vi "Dashboard Main.vi"() -> ()   [LabVIEW 2014]
uses:
  <vilib>/event_ctls.llb/eventvkey.ctl
  <vilib>/Rock Robotics/WPI/Dashboard/WPI_DashboardLogging Global.vi
  <vilib>/Utility/config.llb/Write Key (String).vi
  <vilib>/Utility/config.llb/Write Key (I32).vi
  <vilib>/Utility/config.llb/NI_LVConfig.lvlib
panel:
  in  "TCP":refnum<k5>
  in  "Rec Mode":enum32{"Stop", "Record", "Playback"}(radio)
  in  "Vision":u16(ring) items=["Camera Off", "USB Camera SW", "USB Camera HW", "IP Camera"]
  out "Camera IP":string
  out "Image Message":string="Timeout in Camera Communications"
  in  "Dashboard Tab":T1(tab)
  in  "Camera Settings":T2={"Frame Rate"=30, "Compression"=30, "Size"=1} {"Frame Rate" scale=1.0..30.0; "Size" items=["640x480", "320x240", "160x120"]}
  out "MotorChart R":cluster{"Numeric":dbl, "Numeric":dbl}(graph)
  out "MotorChart L":T3(graph)
  out "MotorSliders R":cluster{"MotorSlide1":dbl, "MotorSlide2":dbl} {"MotorSlide2" scale=-1.0..1.0 scale format="%#_2e"; "MotorSlide1" scale=-1.0..1.0 scale format="%#_2e"}
  out "MotorSliders L":T4 {"MotorSlide4 2" scale=0.0..14.0 scale format="%#_2e"; "MotorSlide2" scale=-1.0..1.0 scale format="%#_2e"; "MotorSlide1" scale=-1.0..1.0 scale format="%#_2e"}
  out "Mode":T5(ring)=enum."Auto Disabled"
  in  "DB Camera Config":bool
  out "fps":dbl format="%#.1g"
  out "Mbps":dbl format="%#.1g"
  out "Mbps 2":bool
  in  "DB/String 9":string
  in  "DB/String 8":string
  in  "DB/String 7":string
  in  "DB/String 6":string
  in  "DB/String 5":string
  in  "DB/String 4":string
  in  "DB/String 3":string
  in  "DB/String 2":string
  in  "DB/String 1":string
  in  "DB/String 0":string
  in  "DB/Slider 0":dbl(slide) scale=0.0..5.0
  in  "DB/Slider 1":dbl(slide) scale=0.0..5.0
  in  "DB/Slider 2":dbl(slide) scale=0.0..5.0
  in  "DB/Slider 3":dbl(slide) scale=0.0..5.0
  out "DB/LED 3":bool
  out "DB/LED 2":bool
  out "DB/LED 1":bool
  out "DB/LED 0":bool
  in  "DB/Button 3":bool
  in  "DB/Button 2":bool
  in  "DB/Button 1":bool
  in  "DB/Button 0":bool caption="New Name"
  in  "Auto Selection":string(combo)
  in  "Test Slider":dbl(slide) scale=0.0..100.0 scale format="%#_3g"
  in  "On/Off":bool caption="Solenoid"
  in  "Test Name":u16(ring) items=["Select the test to run...", "Example Test", "-------------------------------", "List of tests is built in robot code.", "Replace with your own automated tests."]
  in  "Test Tree":string(tree)
  in  "Motor":cluster{"Value":dbl, "Enable":bool} {"Value" scale=-1.0..1.0 scale format="%#_3g"}
  out "Progress":T6 {"Test Progress" scale=0.0..100.0}
  in  "Rev/Fwd":cluster{"Forward":bool, "Reverse":bool}
  in  "Test Ring":u16(ring) items=["Monochrome", "Color"]
  in  "Listbox":i32(listbox)
  out "Tree":string(tree)
  out "Camera Image":T7(plugin-control)
  out "Boolean":bool
  # "Left"
  # "Front"
  # "Right"
  # "Battery"
  # "This tab is a great place for autonomous settings and robot-specific values.\nPlace controls and indicators inside this tab and match name to\nDashboard Variables on robot. You can also delete this comment."
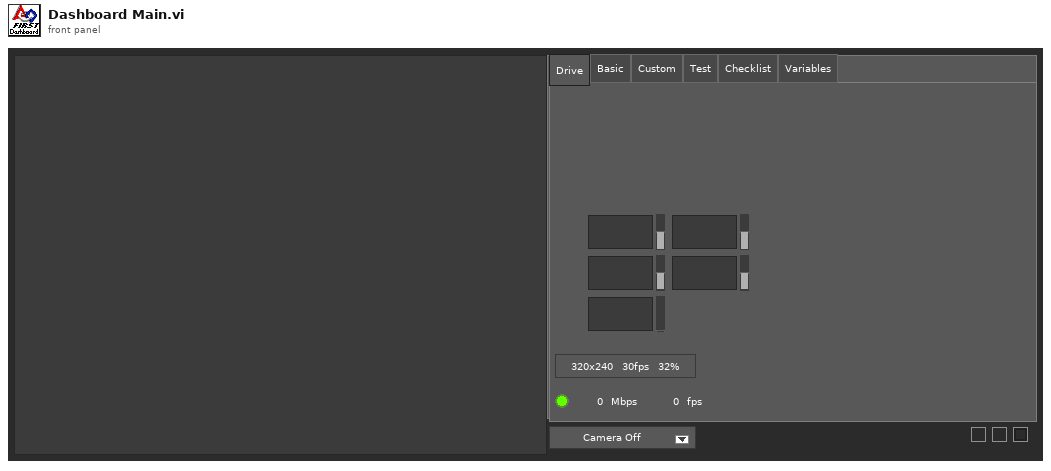
[diagram p1: front panel]
types:
  T1 = enum32{"Drive", "Basic", "Custom", "Test", "Checklist", "Variables"}
  T2 = cluster{"Frame Rate":i32, "Compression":i32, "Size":u16}
  T3 = cluster{"Numeric":dbl, "Numeric":dbl, "Battery V":dbl}
  T4 = cluster{"MotorSlide1":dbl, "MotorSlide2":dbl, "MotorSlide4 2":dbl}
  T5 = enum8{"Tele-Op Disabled", "Tele-Op Enabled", "Auto Disabled", "Auto Enabled", "Test Disabled", "Test Enabled", "Disconnected", "No Code", "E-Stop"}
  T6 = cluster{"Test Progress":u8, "Test Progress Text":string}
  T7 = typedef "IMAQ Image.ctl" = refnum<image>
  T8 = typedef "Image Type" = u32
  T9 = cluster{"Camera Image":refnum<vi>, "Dashboard Tab":refnum<vi>, "Boolean":refnum<vi>, "Vision":refnum<vi>, "Rec Mode":refnum<vi>, "Test Slider":refnum<vi>, "On/Off ":refnum<vi>, "Test Ring":refnum<vi>, "Rev/Fwd":refnum<vi>, "Test Name":refnum<vi>, "Motor":refnum<vi>, "Progress":refnum<vi>, "CheckList":refnum<vi>, "Tree":refnum<vi>, "Test Tree":refnum<vi>}
  T10 = cluster{"Error Strings":string, "Disable Counts":cluster{u16, u16}, "Rail Faults":cluster{u16, u16, u16}, "Robot IP":string, "DB Mode":u8, "Event Info":cluster{"Name":string, "Type":u8, "Number":u16, "Replay":u8}, "Camera Addr":string}
  T11 = cluster{"Storage":cluster{"Disk Free":u64, "RAM Block":u32, "RAM free":u32}, "CPU Utilization":cluster{"CPU % ISR":sgl, "CPU % Time Crit":sgl, "CPU % Timed Str":sgl, "CPU % High":sgl, "CPU % Above":sgl, "CPU % Normal":sgl, "CPU % Low":sgl}, "CAN":cluster{"% Bus Utilization":sgl, "Bus Off Cnt":u32, "TX_FIFO Full Cnt":u32, "Receive Error Cnt":u8, "Transmit Error Cnt":u8}, "HID":cluster{"HID Outputs":u32, "Rumble Low":u16, "Rumble High":u16}[]}
  T12 = cluster{"Status bits":cluster{"Test Mode":bool, "Autonomous":bool, "Enabled":bool, "Code Start":bool, "Brownout":bool, "Reserved 2":bool, "Reserved 3":bool, "E-Stop":bool}, "Code Trace":cluster{"Disabled":bool, "TeleOp":bool, "Auto":bool, "Test":bool}, "Controller Type":enum16{"unknown", "cRIO", "roboRio"}, "Code?":enum16{"unknown", "noCode", "code"}, "Battery V":dbl}
  T13 = cluster{"Control Bits":cluster{"TestMode":bool, "Autonomous":bool, "Enabled":bool, "FMS Present":bool, bool, bool, bool, "E-Stop":bool}, "Team Station ":u8, "Countdown":sgl, "Joystick Values":cluster{"Axes":dbl[], "Buttons":bool[], "POVs":i16[]}[]}
  T14 = cluster{"Axes":dbl[], "Buttons":bool[], "POVs":i16[]}[]
  T15 = cluster{"Axes":dbl[], "Buttons":bool[], "POVs":i16[]}
  T16 = typedef "NI_LVConfig.lvlib/Config Data RefNum.ctl" = refnum<k1>
  T17 = cluster{"Operation":enum16{"Update", "Clear"}, "Color Box":u32}[]
  T18 = typedef "eventvkey.ctl" = enum16{"ASCII", "Enter", "Return", "Shift", "Ctrl", "Alt", "Cmd", "Opt", "Caps", "NumLock", "Clear", "Break", "Up", "Down", "Left", "Right", "Insert", "Delete", "Home", "End", "PageUp", "PageDown", "Escape", "Help", "Pause", "ScrollLock", "F1", "F2", "F3", "F4", "F5", "F6", "F7", "F8", "F9", "F10", "F11", "F12", "F13", "F14", "F15", "F16", "F17", "F18", "F19", "F20", "F21", "F22", "F23", "F24", "Play", "VolumeUp", "VolumeDown", "Mute", "Two Byte Char"}
  T19 = cluster{"Image Size":bool, "Image Type":bool, "Pixel Value":bool, "ROI Information":bool, "Zoom Factor":bool}
  T20 = enum8{"Enabled", "Disabled", "Disabled and Grayed Out"}
  T21 = cluster{"Operation":enum16{"Update", "Clear"}, "Color Box":u32}
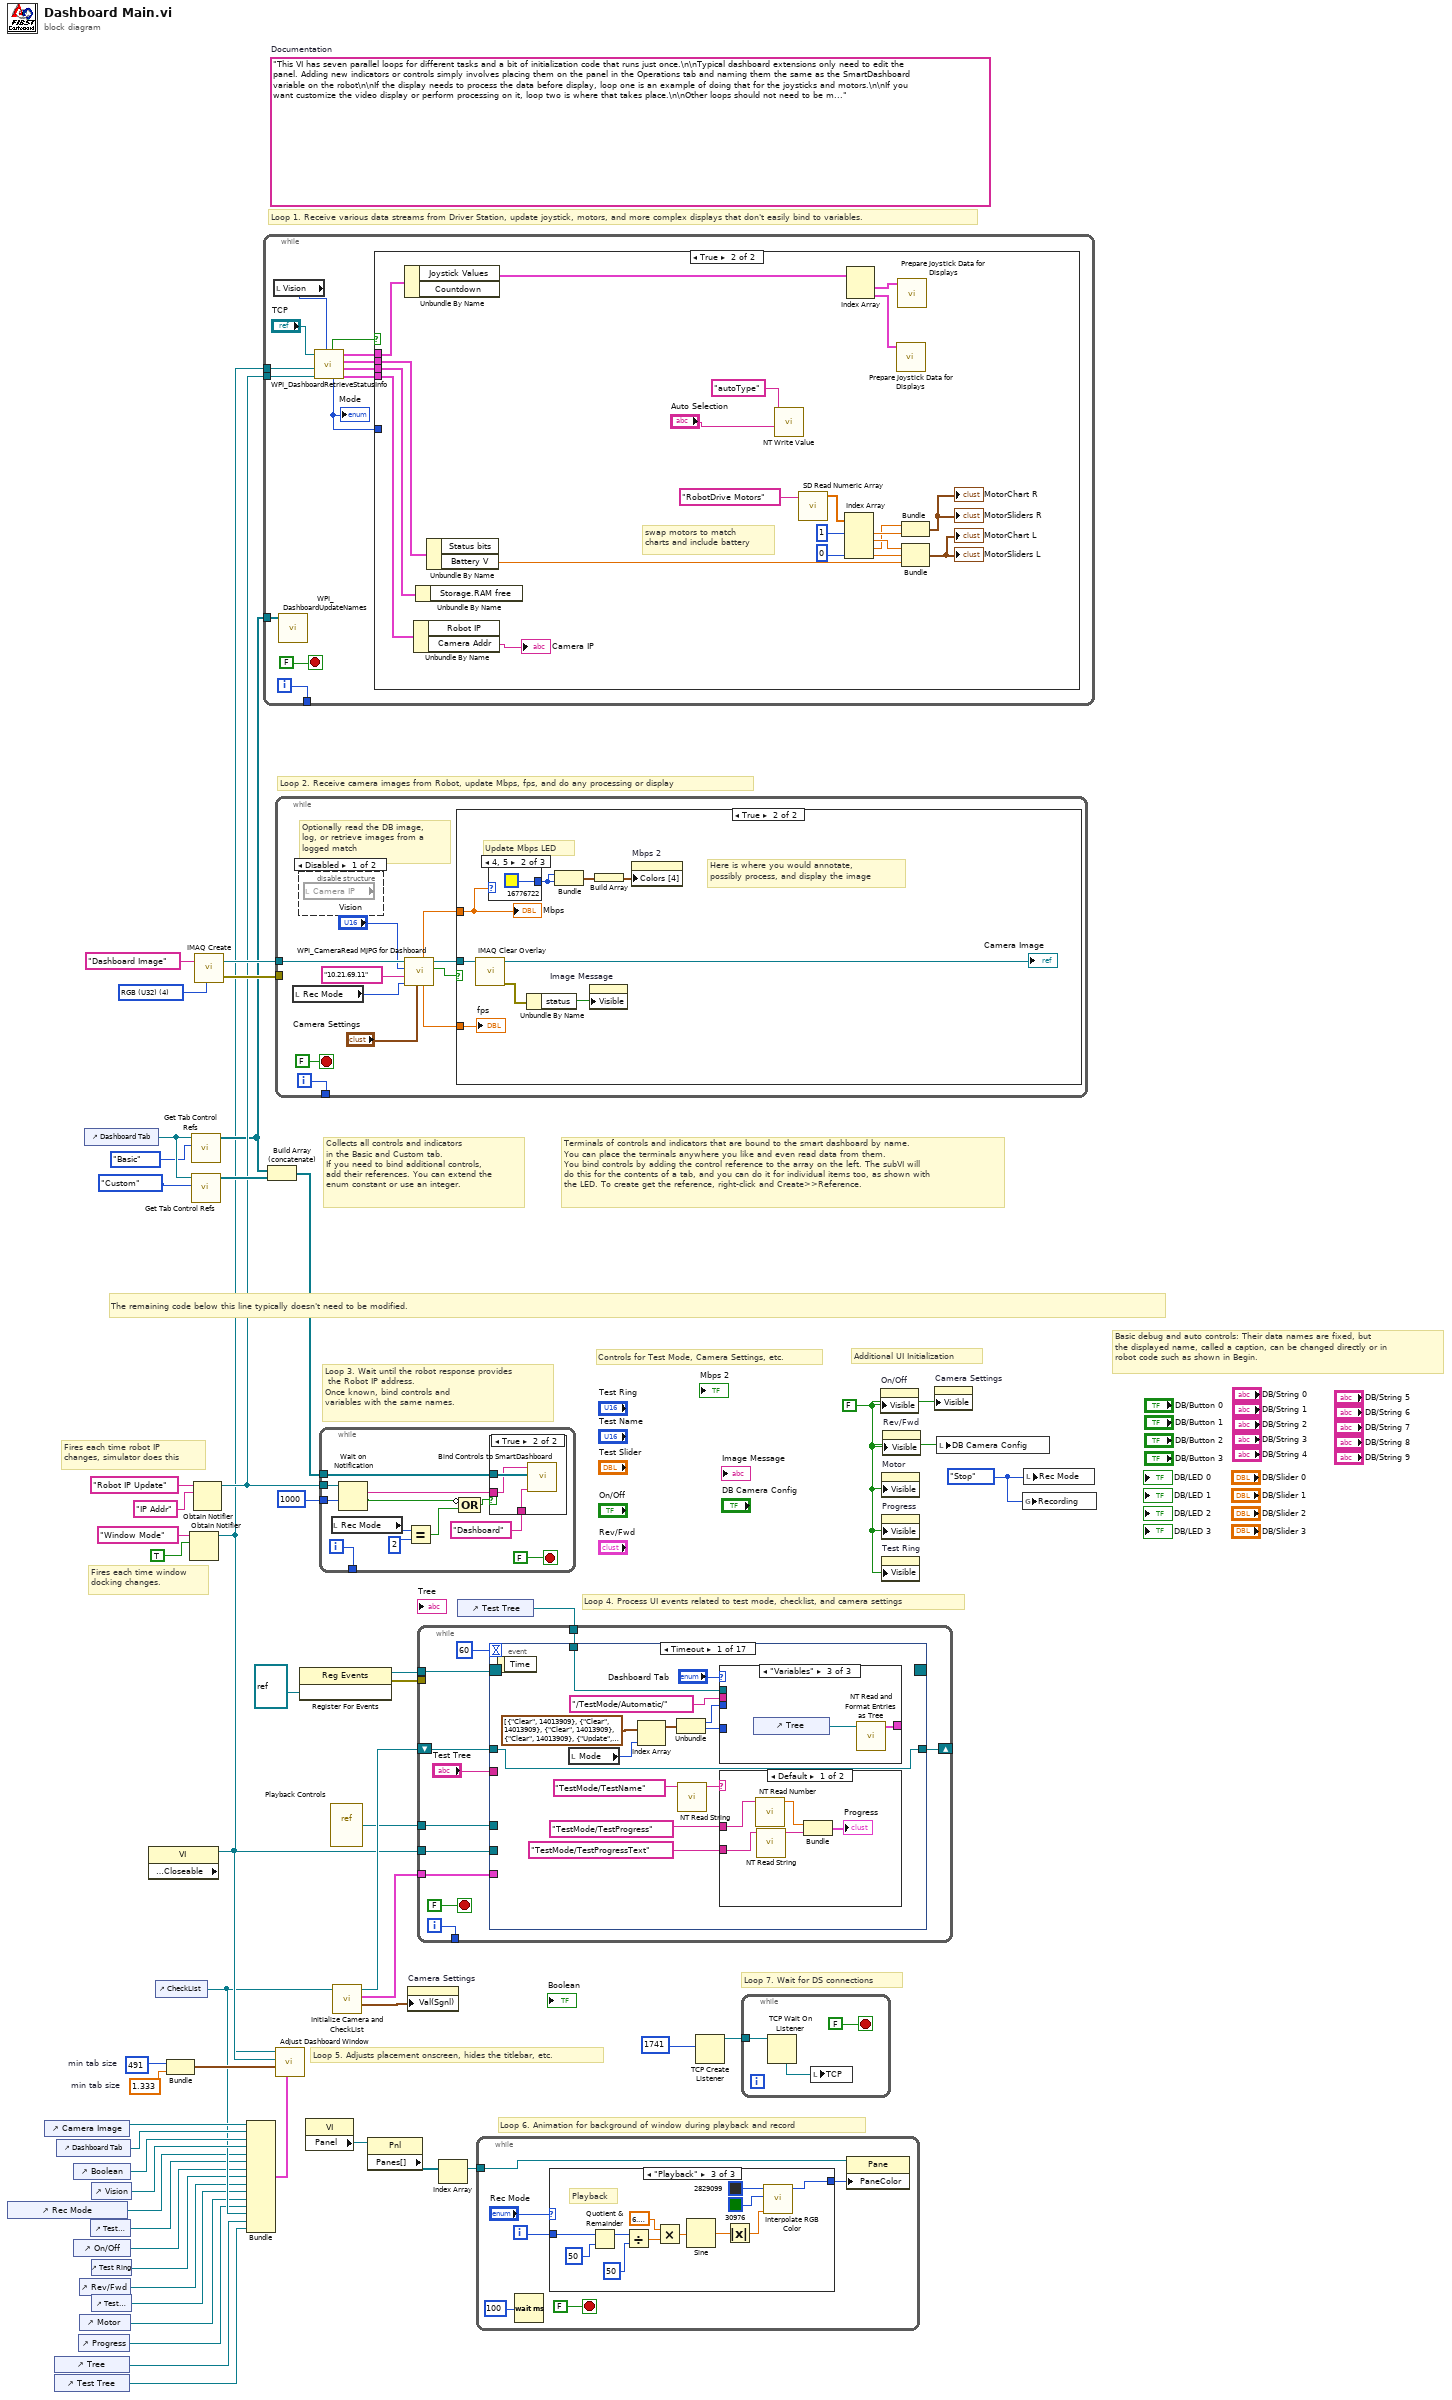
[diagram p0: block diagram]
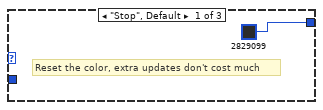
[diagram p3: hidden frame]
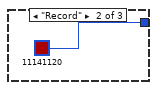
[diagram p4: hidden frame]
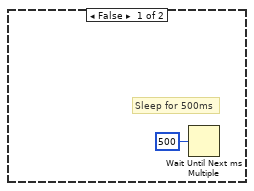
[diagram p7: hidden frame]
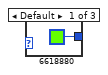
[diagram p8: hidden frame]
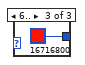
[diagram p9: hidden frame]
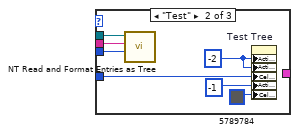
[diagram p11: hidden frame]
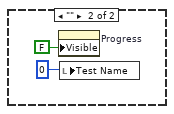
[diagram p12: hidden frame]
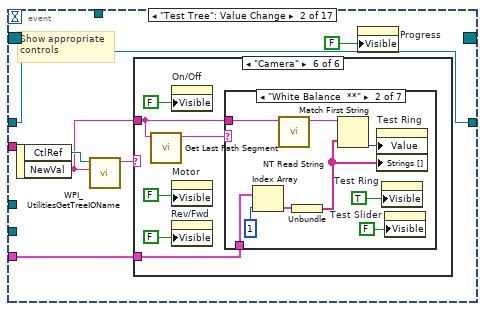
[diagram p13: hidden frame]
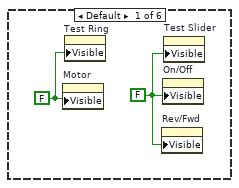
[diagram p14: hidden frame]
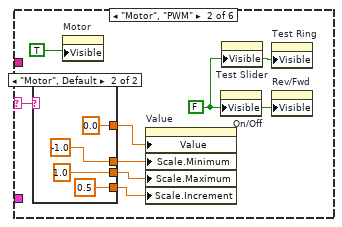
[diagram p15: hidden frame]
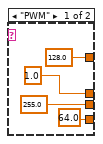
[diagram p16: hidden frame]
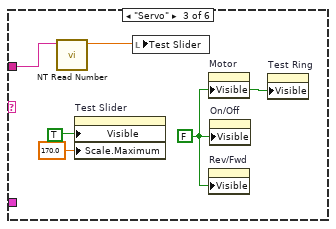
[diagram p17: hidden frame]
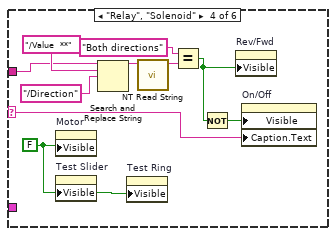
[diagram p18: hidden frame]
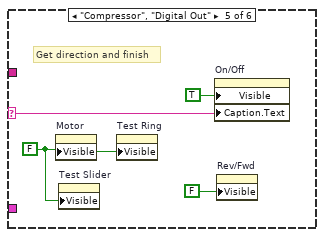
[diagram p19: hidden frame]
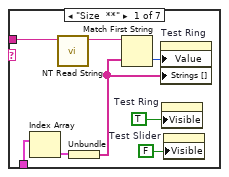
[diagram p20: hidden frame]
diagram:
  w24 = 491  # min tab size
  w23 = 1.333  # min tab size
  w32 = enum32{"Stop", "Record", "Playback"}."Stop" ("Rec Mode")
  w6 = FALSE ("Visible")
  (unwired) "This VI has seven parallel loops for different tasks and a bit of initialization code that runs just once.\n\nTypical dashboard extensions only need to edit the panel. Adding new indicators or controls simply involves placing them on the panel in the Operations tab and naming them the same as the SmartDashboard variable on the robot\n\nIf the display needs to process the data before display, loop one is an example of doing that for the joysticks and motors.\n\nIf you want customize the video display or perform processing on it, loop two is where that takes place.\n\nOther loops should not need to be modified. They are pretty standard, and document the task they perform."  # Documentation
  w52 = T8 4 items=["Grayscale (U8)", "Grayscale (I16)", "Grayscale (SGL)", "Complex (CSG)", "RGB (U32)", "HSL (U32)", "RGB (U64)"] ("Image Type")
  # "Loop 7. Wait for DS connections"
  # "Basic debug and auto controls: Their data names are fixed, but\nthe displayed name, called a caption, can be changed directly or in\nrobot code such as shown in Begin."
  # "Controls for Test Mode, Camera Settings, etc."
  # "Additional UI Initialization"
  # "Loop 6. Animation for background of window during playback and record"
  # "Fires each time robot IP\nchanges, simulator does this"
  # "Fires each time window\ndocking changes."
  # "Collects all controls and indicators\nin the Basic and Custom tab.\nIf you need to bind additional controls,\nadd their references. You can extend the\nenum constant or use an integer."
  # "The remaining code below this line typically doesn't need to be modified."
  # "Loop 4. Process UI events related to test mode, checklist, and camera settings"
  # "Terminals of controls and indicators that are bound to the smart dashboard by name.\nYou can place the terminals anywhere you like and even read data from them.\nYou bind controls by adding the control reference to the array on the left. The subVI will\ndo this for the contents of a tab, and you can do it for individual items too, as shown with\nthe LED. To create get the reference, right-click and Create>>Reference."
  # "Loop 3. Wait until the robot response provides\n the Robot IP address.\nOnce known, bind controls and\nvariables with the same names."
  # "Loop 5. Adjusts placement onscreen, hides the titlebar, etc."
  # "Loop 1. Receive various data streams from Driver Station, update joystick, motors, and more complex displays that don't easily bind to variables."
  # "Loop 2. Receive camera images from Robot, update Mbps, fps, and do any processing or display"
  n1 = control-ref of="Rec Mode"() -> (w12:refnum<vi>)
  n2 = control-ref of="Camera Image"() -> (w27:refnum<vi>)
  n3 = control-ref of="Tree"() -> (w16:refnum<vi>)
  n4 = control-ref of="Test Tree"() -> (w15:refnum<vi>)
  n5 = control-ref of="Dashboard Tab"() -> (w26:refnum<vi>)
  n6 = control-ref of="Boolean"() -> (w21:refnum<vi>)
  n7 = control-ref of="On/Off"() -> (w10:refnum<vi>)
  n8 = control-ref of="Progress"() -> (w7:refnum<vi>)
  n9 = control-ref of="Rev/Fwd"() -> (w8:refnum<vi>)
  n10 = control-ref of="Motor"() -> (w13:refnum<vi>)
  n11 = control-ref of="Dashboard Tab"() -> (w30:refnum<vi>)
  n12 = control-ref of="Test Slider"() -> (w11:refnum<vi>)
  n13 = control-ref of="Vision"() -> (w25:refnum<vi>)
  n14 = control-ref of="Test Ring"() -> (w9:refnum<vi>)
  n15 = control-ref of="Test Name"() -> (w14:refnum<vi>)
  n16 = property class="VI" props=["Front Panel.Closeable"]() -> (reference out=w31:refnum<vi>)  [unwired: 2 in, 2 out]
  n17 = control-ref of="CheckList"() -> (w17:refnum<vi>)
  n18 = Bundle("min tab size"=w24, "min tab size"=w23) -> (w22:cluster{"min tab size":i32, "min tab size":dbl})  [unwired: 1 in]
  n19 = Obtain Notifier(name (unnamed)="Window Mode", notification data type=TRUE) -> (notifier out=w3:refnum<notifier>)  [unwired: 2 in, 2 out]
  n20 = call <vilib>:"Get Tab Control Refs.vi"("Page Index"=T1."Basic" ("Dashboard Tab"), "TabControl in"=w30) -> ("ControlsOnPage"=w4:refnum<vi>[])  [unwired: 9 in]
  n21 = call <vilib>:"Get Tab Control Refs.vi"("Page Index"=T1."Custom" ("Dashboard Tab"), "TabControl in"=w30) -> ("ControlsOnPage"=w29:refnum<vi>[])  [unwired: 9 in]
  n22 = Obtain Notifier(name (unnamed)="Robot IP Update", notification data type="IP Addr" ("name (unnamed)")) -> (notifier out=w5:refnum<notifier>)  [unwired: 2 in, 2 out]
  n23 = call "IMAQ Create"("Image Name"="Dashboard Image", "Image Type"=w52) -> ("New Image"=w50:T7, "error out"=w49:errorcluster)  [unwired: 2 in, 1 out]
  n24 = Bundle("Camera Image"=w27, "Dashboard Tab"=w26, "Boolean"=w21, "Vision"=w25, "Rec Mode"=w12, "Test Slider"=w11, "On/Off"=w10, "Test Ring"=w9, "Rev/Fwd"=w8, "Test Name"=w14, "Motor"=w13, "Progress"=w7, "CheckList"=w17, "Tree"=w16, "Test Tree"=w15) -> (w18:T9)  [unwired: 1 in]
  n25 = while {
    tunnel: [w64] -> _
    tunnel: w5 -> [w58]
    tunnel: w4 -> [w57]
    tunnel: w3 -> [w53]
    i -> [w64]
    stop <- FALSE stop-if-true
    n26 = local read "Vision"() -> (w55:u16)
    n27 = call <vilib>:"WPI_DashboardUpdateNames.vi"("Controls on Tab"=w57) -> ()  [unwired: 11 in]
    n28 = call <vilib>:"WPI_DashboardRetrieveStatusInfo.vi"("Vision"=w55, "Binding Refnum"=w58, "Window Mode Notifier"=w53, "TCP Cnx"="TCP") -> ("Power and Errors"=w59:T10, "Robot Metrics"=w62:T11, "Status Info"=w63:T12, "Control Info"=w60:T13, "Robot Mode"=w56:T5, "Process?"=w61:bool)  [unwired: 2 in]
    "Mode" <- w56
    n29 = case shown="True" w61 {
      tunnel: w63 -> [_ w86]
      tunnel: w62 -> [_ w85]
      tunnel: w60 -> [_ w84]
      tunnel: w59 -> [_ w83]
      tunnel: w56 -> [_ _]
      frame False {
      }
      frame True {
        # "swap motors to match\ncharts and include battery"
        n30 = Unbundle By Name(w84) -> ("Joystick Values"=w71:T14)  [unwired: 1 out]
        n31 = Unbundle By Name(w83) -> ("Camera Addr"=→"Camera IP":string)  [unwired: 1 out]
        n32 = Unbundle By Name(w85) -> ()  [unwired: 1 out]
        n33 = Unbundle By Name(w86) -> ("Battery V"=w72:dbl)  [unwired: 1 out]
        n34 = call-poly <vilib>:"NT Write Value.vi"("String"="Auto Selection", "Name"="autoType") -> ()  [unwired: 9 in, 1 out]
        n35 = call <vilib>:"SD Read Numeric Array.vi"("Name"="RobotDrive Motors") -> ("Numeric Array"=w74:dbl[])  [unwired: 8 in, 2 out]
        n36 = Index Array(array=w74, index #1=1, index #4=0) -> (element #1=w78:dbl, element #2=w79:dbl, element #3=w77:dbl, element #4=w82:dbl)  [unwired: 2 in]
        n37 = Index Array(array=w71) -> (element #1=w70:T15, element #2=w68:T15)  [unwired: 2 in]
        n38 = call "Prepare Joystick Data for Displays.vi"("Joystick Values"=w68) -> ()  [unwired: 8 in, 3 out]
        n39 = call "Prepare Joystick Data for Displays.vi"("Joystick Values"=w70) -> ()  [unwired: 8 in, 3 out]
        n40 = Bundle("Numeric"=w77, "Numeric"=w78) -> (→"MotorChart R" →"MotorSliders R":cluster{"Numeric":dbl, "Numeric":dbl})  [unwired: 1 in]
        n41 = Bundle("Numeric"=w79, "Numeric"=w82, "Battery V"=w72) -> (→"MotorChart L" →"MotorSliders L":T3)  [unwired: 1 in]
      }
    }
  }
  n42 = Build Array (concatenate)(w4, w29) -> (w28:refnum<vi>[])
  n43 = while {
    tunnel: w50 -> [w95]
    tunnel: w49 -> [_]
    tunnel: [w96] -> _
    i -> [w96]
    stop <- FALSE stop-if-true
    # "Optionally read the DB image,\nlog, or retrieve images from a\nlogged match"
    n44 = local read "Rec Mode"() -> (w89:enum32{"Stop", "Record", "Playback"})
    n45 = disable-structure shown="Disabled" {
      frame Disabled {
        n46 = local read "Camera IP"() -> ()  [unwired: 1 out]
      }
      frame Enabled {
      }
    }
    n47 = call <vilib>:"WPI_CameraRead MJPG for Dashboard.vi"("Camera Settings"="Camera Settings", "Rec Mode"=w89, "Camera IP"="10.21.69.11", "Camera Mode"="Vision", "Refnum in"=w95) -> ("Active"=w93:bool, "Refnum out"=w94:T7, "FPS"=w92:dbl, "Bandwidth (Mbps)"=w91:dbl)  [unwired: 3 in]
    n48 = case shown="True" w93 {
      tunnel: w94 -> [_ w102]
      tunnel: w91 -> [_ w101]
      tunnel: w92 -> [_ w99]
      frame False {
        # "Sleep for 500ms"
        n49 = Wait Until Next ms Multiple(millisecond multiple=u32 500) -> ()  [unwired: 1 out]
      }
      frame True {
        # "Here is where you would annotate,\npossibly process, and display the image"
        # "Update Mbps LED"
        n50 = call "IMAQ Clear Overlay"("Image"=w102) -> ("error out"=w106:errorcluster, "Image Out"=→"Camera Image":T7)  [unwired: 2 in, 7 out]
        n51 = case shown="4, 5" w101 {
          tunnel: [u32 6618880 ("Color Box") u32 16776722 ("Color Box") u32 16716800 ("Color Box")] -> w103
          frame Default {
          }
          frame 4, 5 {
          }
          frame 6.. {
          }
        }
        n52 = Unbundle By Name(w106) -> ("status"=w107:bool)
        n53 = Bundle("Color Box"=w103, "Color Box"=w103) -> (w105:cluster{"Color Box":u32, "Color Box":u32})  [unwired: 1 out]
        n54 = property on="Image Message" class="Str"("Visible"=w107) -> ()  [unwired: 2 in, 2 out]
        n55 = Build Array(w105) -> (w104:cluster{"Color Box":u32, "Color Box":u32}[])
        n56 = property on="Mbps 2" class="Bool (strict)"("Colors [4]"=w104) -> ()  [unwired: 2 in, 2 out]
        "Mbps" <- w101
        "fps" <- w99
      }
    }
  }
  n57 = call "Adjust Dashboard Window.vi"("Sizing Refnums"=w18, "Size Constraints"=w22, "VI"=w31, "Notifier in"=w3) -> ()  [unwired: 8 in]
  n58 = register-events(refnum<vi> refnum) -> (reference out=w36:refnum<event-registration>, error out=w35:errorcluster)  [unwired: 2 in]
  n59 = property class="VI"() -> ("Panel"=w39:refnum<vi>)  [unwired: 2 in, 2 out]
  n60 = while {
    tunnel: w28 -> [w122]
    tunnel: w5 -> [w120]
    tunnel: [w118] -> _
    tunnel: u32 1000 ("milliseconds to wait") -> [w117]
    i -> [w118]
    stop <- FALSE stop-if-true
    n61 = local read "Rec Mode"() -> (w113:enum32{"Stop", "Record", "Playback"})
    n62 = Wait on Notification(notifier=w120, timeout in ms (-1)=w117) -> (notification=w119:string, timed out?=w115:bool)  [unwired: 2 in, 2 out]
    n63 = Equal?(x=w113, y=u16 2 ("Rec Mode")) -> (x = y?=w114:bool)
    n64 = Compound Arithmetic op=OR(invert w115, w114) -> (w116:bool)
    n65 = case shown="True" w116 {
      tunnel: w122 -> [_ w125]
      tunnel: w119 -> [_ w124]
      tunnel: "Dashboard" -> [_ w123]
      frame False {
      }
      frame True {
        n66 = call <vilib>:"Bind Controls to SmartDashboard.vi"("Client Name"=w123, "Bound Control Refs"=w125, "Server IP Address"=w124) -> ()  [unwired: 9 in]
      }
    }
  }
  n67 = vi-ref "Playback Controls.vi"() -> (w37:refnum<vi>)
  n68 = call "Initialize Camera and CheckList.vi"("ListBox in"=w17) -> ("Cluster"=w43:cluster{"value":i32, "value":i32, "index":i32}, "Array"=w44:cluster{string[]}[], "File Refnum"=w42:T16)  [unwired: 8 in]
  n69 = property class="Pnl"(reference=w39) -> ("Panes[]"=w40:refnum<vi>[])  [unwired: 1 in, 2 out]
  n70 = property on="Camera Settings" class="Clust (strict)"("Val(Sgnl)"=w43) -> ()  [unwired: 2 in, 2 out]
  n71 = Index Array(array=w40) -> (element=w38:refnum<vi>)  [unwired: 1 in]
  n72 = control-ref of="Test Tree"() -> (w41:refnum<vi>)
  n73 = while {
    tunnel: w44 -> [w133]
    shift-right: [w132] -> _
    shift-left: w42 -> [w131]
    tunnel: [w130] -> _
    tunnel: w41 -> [w129]
    tunnel: w37 -> [w128]
    tunnel: w36 -> [w127]
    tunnel: w35 -> [_]
    tunnel: w31 -> [w126]
    i -> [w130]
    stop <- FALSE stop-if-true
    n74 = event shown="[0] Timeout" {
      selector: w127 -> [_ _ _ _ _ _ _ _ _ _ _ _ _ _ _ _ _]
      dyn-events: [_ _ _ _ _ _ _ _ _ _ _ _ _ w371 _ _ _] -> _
      timeout: u32 60 ("milliseconds to wait") -> [_ _ _ _ _ _ _ _ _ _ _ _ _ _ _ _ _]
      tunnel: w129 -> [w145 _ _ _ _ _ _ _ _ _ _ _ _ _ _ _ _]
      tunnel: "Test Tree" -> [_ _ _ _ _ _ _ _ w340 w348 w350 w354 w362 _ _ _ _]
      tunnel: w133 -> [_ w167 _ _ _ _ w304 w334 _ _ _ _ _ _ _ _ _]
      tunnel: [w141 w166 w265 w270 w278 w290 w303 w327 w339 w346 w349 w353 w361 w373 w387 w388 w398] -> w132
      tunnel: w131 -> [w141 w166 w265 w270 w278 w290 w302 w327 w339 w346 w349 w353 w361 w373 w387 w388 w398]
      tunnel: w128 -> [_ _ _ _ _ _ _ _ _ _ _ _ _ w374 _ w391 _]
      tunnel: w126 -> [_ _ _ _ _ _ _ _ _ _ _ _ _ w369 _ _ _]
      event Timeout {
        n75 = event-data() -> ()  [unwired: 1 in, 1 out]
        n76 = local read "Mode"() -> (w144:T5)
        n77 = Index Array(array=T17 [{"Operation"=enum."Clear", "Color Box"=14013909}, {"Operation"=enum."Clear", "Color Box"=14013909}, {"Operation"=enum."Clear", "Color Box"=14013909}, {"Operation"=enum."Clear", "Color Box"=14013909}, {"Operation"=enum."Update", "Color Box"=14013909}, {"Operation"=enum."Update", "Color Box"=16777215}, {"Operation"=enum."Clear", "Color Box"=14013909}, {"Operation"=enum."Clear", "Color Box"=14013909}, {"Operation"=enum."Clear", "Color Box"=14013909}], index=w144) -> (element=w139:T21)
        n78 = Unbundle(w139) -> ("Operation"=w138:enum16{"Update", "Clear"}, "Color Box"=w137:u32)
        n79 = call <vilib>:"NT Read String.vi"("Name"="TestMode/TestName") -> ("String"=w148:string)  [unwired: 9 in, 1 out]
        n80 = case shown="\"Variables\"" "Dashboard Tab" {
          tunnel: w145 -> [_ w156 _]
          tunnel: "/TestMode/Automatic/" ("Name Pattern") -> [_ w155 _]
          tunnel: w138 -> [_ w154 _]
          tunnel: [_ _ w158] -> _
          tunnel: w137 -> [_ w150 _]
          frame "Custom", Default {
          }
          frame "Test" {
            w153 = -2 ("Active Item:Row Number")
            n81 = call <vilib>:"NT Read and Format Entries as Tree.vi"("Operation"=w154, "Name Pattern"=w155, "Tree Refnum"=w156) -> ()  [unwired: 7 in, 2 out]
            n82 = property on="Test Tree" class="Tree (strict)"("Active Item Row Number"=w153, "ActiveColNum"=w153, "CellBG"=w150, "Active Item Row Number"=-1 ("Active Item:Row Number"), "CellBG"=u32 5789784 ("Color Box")) -> ()  [unwired: 2 in, 2 out]
          }
          frame "Variables" {
            n83 = control-ref of="Tree"() -> (w157:refnum<vi>)
            n84 = call <vilib>:"NT Read and Format Entries as Tree.vi"("Tree Refnum"=w157) -> ("Formatted Strings"=w158:cluster{"Name":string, "Value":string}[])  [unwired: 9 in, 1 out]
          }
        }
        n85 = case shown="Default" w148 {
          tunnel: "TestMode/TestProgress" ("Name") -> [w160 _]
          tunnel: "TestMode/TestProgressText" ("Name") -> [w159 _]
          frame Default {
            n86 = call <vilib>:"NT Read Number.vi"("Name"=w160) -> ("Numeric"=w161:dbl)  [unwired: 9 in, 1 out]
            n87 = call <vilib>:"NT Read String.vi"("Name"=w159) -> ("String"=w162:string)  [unwired: 9 in, 1 out]
            n88 = Bundle("Numeric"=w161, "String"=w162) -> (→"Progress":cluster{"Numeric":dbl, "String":string})  [unwired: 1 in]
          }
          frame "" {
            n89 = property on="Progress" class="Clust (strict)"("Visible"=FALSE) -> ()  [unwired: 2 in, 2 out]
            n90 = local write "Test Name"(u16 0) -> ()
          }
        }
      }
      event "Test Tree": Value Change {
        # "Show appropriate\ncontrols"
        n91 = event-data() -> ("CtlRef"=w170:refnum<vi>, "NewVal"=w168:string)  [unwired: 1 in]
        n92 = call <vilib>:"WPI_UtilitiesGetTreeIOName.vi"("NewVal"=w168, "TreeControl in"=w170) -> ("I/O Name"=w171:string)  [unwired: 9 in]
        n93 = case shown="\"Camera\"" w171 {
          selector: w171 -> [_ w178 _ w196 w205 _]
          tunnel: w168 -> [_ _ w193 w195 _ w212]
          tunnel: w167 -> [_ _ _ _ _ w211]
          frame Default {
            w173 = FALSE ("Visible")
            w172 = FALSE ("Visible")
            n94 = property on="Motor" class="Clust (strict)"("Visible"=w172) -> ()  [unwired: 2 in, 2 out]
            n95 = property on="Test Ring" class="Ring (strict)"("Visible"=w172) -> ()  [unwired: 2 in, 2 out]
            n96 = property on="Rev/Fwd" class="Clust (strict)"("Visible"=w173) -> ()  [unwired: 2 in, 2 out]
            n97 = property on="On/Off" class="Bool (strict)"("Visible"=w173) -> ()  [unwired: 2 in, 2 out]
            n98 = property on="Test Slider" class="Slide (strict)"("Visible"=w173) -> ()  [unwired: 2 in, 2 out]
          }
          frame "Motor", "PWM" {
            w179 = FALSE ("Visible")
            n99 = case shown="\"Motor\", Default" w178 {
              tunnel: [1.0 ("Value") -1.0 ("Value")] -> w177
              tunnel: [255.0 ("Value") 1.0 ("Value")] -> w176
              tunnel: [128.0 ("Value") 0.0 ("Value")] -> w175
              tunnel: [64.0 ("Value") 0.5 ("Value")] -> w174
              frame "PWM" {
              }
              frame "Motor", Default {
              }
            }
            n100 = property on="Motor" class="Clust (strict)"("Visible"=TRUE) -> ()  [unwired: 2 in, 2 out]
            n101 = property on="Value" class="Slide (strict)"("Value"=w175, "Scale.Minimum"=w177, "Scale.Maximum"=w176, "Scale.Increment"=w174) -> ()  [unwired: 2 in, 2 out]
            n102 = property on="On/Off" class="Bool (strict)"("Visible"=w179) -> ()  [unwired: 2 in, 2 out]
            n103 = property on="Test Slider" class="Slide (strict)"("Visible"=w179) -> ()  [unwired: 2 in, 2 out]
            n104 = property on="Test Ring" class="Ring (strict)"("Visible"=w179) -> ()  [unwired: 2 in, 2 out]
            n105 = property on="Rev/Fwd" class="Clust (strict)"("Visible"=w179) -> ()  [unwired: 2 in, 2 out]
          }
          frame "Servo" {
            w191 = FALSE ("Visible")
            n106 = call <vilib>:"NT Read Number.vi"("Name"=w193) -> ("Numeric"=w192:dbl)  [unwired: 9 in, 1 out]
            n107 = property on="Test Slider" class="Slide (strict)"("Visible"=TRUE, "Scale.Maximum"=170.0 ("Scale.Range:Maximum")) -> ()  [unwired: 2 in, 2 out]
            n108 = local write "Test Slider"(w192) -> ()
            n109 = property on="Motor" class="Clust (strict)"("Visible"=w191) -> ()  [unwired: 2 in, 2 out]
            n110 = property on="Rev/Fwd" class="Clust (strict)"("Visible"=w191) -> ()  [unwired: 2 in, 2 out]
            n111 = property on="On/Off" class="Bool (strict)"("Visible"=w191) -> ()  [unwired: 2 in, 2 out]
            n112 = property on="Test Ring" class="Ring (strict)"("Visible"=w191) -> ()  [unwired: 2 in, 2 out]
          }
          frame "Relay", "Solenoid" {
            w194 = FALSE ("Visible")
            n113 = property on="Motor" class="Clust (strict)"("Visible"=w194) -> ()  [unwired: 2 in, 2 out]
            n114 = property on="Test Slider" class="Slide (strict)"("Visible"=w194) -> ()  [unwired: 2 in, 2 out]
            n115 = Search and Replace String(input string=w195, search string="/Value  **", replace string="/Direction") -> (result string=w201:string)  [unwired: 5 in, 3 out]
            n116 = property on="Test Ring" class="Ring (strict)"("Visible"=w194) -> ()  [unwired: 2 in, 2 out]
            n117 = call <vilib>:"NT Read String.vi"("Name"=w201) -> ("String"=w199:string)  [unwired: 9 in, 1 out]
            n118 = Equal?(x="Both directions", y=w199) -> (x = y?=w197:bool)
            n119 = Not(x=w197) -> (.not. x?=w198:bool)
            n120 = property on="Rev/Fwd" class="Clust (strict)"("Visible"=w197) -> ()  [unwired: 2 in, 2 out]
            n121 = property on="On/Off" class="Bool (strict)"("Visible"=w198, "Caption.Text"=w196) -> ()  [unwired: 2 in, 2 out]
          }
          frame "Compressor", "Digital Out" {
            w204 = FALSE ("Visible")
            # "Get direction and finish"
            n122 = property on="Motor" class="Clust (strict)"("Visible"=w204) -> ()  [unwired: 2 in, 2 out]
            n123 = property on="Test Slider" class="Slide (strict)"("Visible"=w204) -> ()  [unwired: 2 in, 2 out]
            n124 = property on="Test Ring" class="Ring (strict)"("Visible"=w204) -> ()  [unwired: 2 in, 2 out]
            n125 = property on="On/Off" class="Bool (strict)"("Visible"=TRUE, "Caption.Text"=w205) -> ()  [unwired: 2 in, 2 out]
            n126 = property on="Rev/Fwd" class="Clust (strict)"("Visible"=FALSE) -> ()  [unwired: 2 in, 2 out]
          }
          frame "Camera" {
            n127 = call <vilib>:"Get Last Path Segment.vi"("String in"=w212) -> ("String out"=w213:string)  [unwired: 10 in]
            n128 = property on="On/Off" class="Bool (strict)"("Visible"=FALSE) -> ()  [unwired: 2 in, 2 out]
            n129 = property on="Motor" class="Clust (strict)"("Visible"=FALSE) -> ()  [unwired: 2 in, 2 out]
            n130 = property on="Rev/Fwd" class="Clust (strict)"("Visible"=FALSE) -> ()  [unwired: 2 in, 2 out]
            n131 = case shown="\"White Balance  **\"" w213 {
              tunnel: w212 -> [w219 w228 w237 w246 w255 _ w261]
              tunnel: w211 -> [w217 w225 w234 w243 w252 _ _]
              frame "Size  **" {
                n132 = Index Array(array=w217) -> (element=w216:cluster{string[]})  [unwired: 1 in]
                n133 = call <vilib>:"NT Read String.vi"("Name"=w219) -> ("String"=w218:string)  [unwired: 9 in, 1 out]
                n134 = Unbundle(w216) -> (w214:string[])
                n135 = Match First String(2:w214, 3:w218) -> (0:w215:i32)  [unwired: 1 out]
                n136 = property on="Test Ring" class="Ring (strict)"("Value"=w215, "Strings []"=w214) -> ()  [unwired: 2 in, 2 out]
                n137 = property on="Test Ring" class="Ring (strict)"("Visible"=TRUE) -> ()  [unwired: 2 in, 2 out]
                n138 = property on="Test Slider" class="Slide (strict)"("Visible"=FALSE) -> ()  [unwired: 2 in, 2 out]
              }
              frame "White Balance  **" {
                n139 = Index Array(array=w225, index=1) -> (element=w226:cluster{string[]})
                n140 = call <vilib>:"NT Read String.vi"("Name"=w228) -> ("String"=w227:string)  [unwired: 9 in, 1 out]
                n141 = Unbundle(w226) -> (w223:string[])
                n142 = Match First String(2:w223, 3:w227) -> (0:w222:i32)  [unwired: 1 out]
                n143 = property on="Test Ring" class="Ring (strict)"("Value"=w222, "Strings []"=w223) -> ()  [unwired: 2 in, 2 out]
                n144 = property on="Test Ring" class="Ring (strict)"("Visible"=TRUE) -> ()  [unwired: 2 in, 2 out]
                n145 = property on="Test Slider" class="Slide (strict)"("Visible"=FALSE) -> ()  [unwired: 2 in, 2 out]
              }
              frame "Exposure  **" {
                n146 = Index Array(array=w234, index=2) -> (element=w235:cluster{string[]})
                n147 = call <vilib>:"NT Read String.vi"("Name"=w237) -> ("String"=w236:string)  [unwired: 9 in, 1 out]
                n148 = Unbundle(w235) -> (w231:string[])
                n149 = Match First String(2:w231, 3:w236) -> (0:w232:i32)  [unwired: 1 out]
                n150 = property on="Test Ring" class="Ring (strict)"("Value"=w232, "Strings []"=w231) -> ()  [unwired: 2 in, 2 out]
                n151 = property on="Test Ring" class="Ring (strict)"("Visible"=TRUE) -> ()  [unwired: 2 in, 2 out]
                n152 = property on="Test Slider" class="Slide (strict)"("Visible"=FALSE) -> ()  [unwired: 2 in, 2 out]
              }
              frame "Exposure Priority  **" {
                n153 = Index Array(array=w243, index=3) -> (element=w244:cluster{string[]})
                n154 = call <vilib>:"NT Read String.vi"("Name"=w246) -> ("String"=w245:string)  [unwired: 9 in, 1 out]
                n155 = Unbundle(w244) -> (w240:string[])
                n156 = Match First String(2:w240, 3:w245) -> (0:w241:i32)  [unwired: 1 out]
                n157 = property on="Test Ring" class="Ring (strict)"("Value"=w241, "Strings []"=w240) -> ()  [unwired: 2 in, 2 out]
                n158 = property on="Test Ring" class="Ring (strict)"("Visible"=TRUE) -> ()  [unwired: 2 in, 2 out]
                n159 = property on="Test Slider" class="Slide (strict)"("Visible"=FALSE) -> ()  [unwired: 2 in, 2 out]
              }
              frame "Color Enable  **" {
                n160 = Index Array(array=w252, index=4) -> (element=w253:cluster{string[]})
                n161 = call <vilib>:"NT Read String.vi"("Name"=w255) -> ("String"=w254:string)  [unwired: 9 in, 1 out]
                n162 = Unbundle(w253) -> (w249:string[])
                n163 = Match First String(2:w249, 3:w254) -> (0:w250:i32)  [unwired: 1 out]
                n164 = property on="Test Ring" class="Ring (strict)"("Value"=w250, "Strings []"=w249) -> ()  [unwired: 2 in, 2 out]
                n165 = property on="Test Ring" class="Ring (strict)"("Visible"=TRUE) -> ()  [unwired: 2 in, 2 out]
                n166 = property on="Test Slider" class="Slide (strict)"("Visible"=FALSE) -> ()  [unwired: 2 in, 2 out]
              }
              frame Default {
                n167 = property on="Test Ring" class="Ring (strict)"("Visible"=FALSE) -> ()  [unwired: 2 in, 2 out]
                n168 = property on="Test Slider" class="Slide (strict)"("Visible"=FALSE) -> ()  [unwired: 2 in, 2 out]
              }
              frame "Brightness  **", "Color Level  **", "Compression  **", "FPS  **", "Sharpness  **" {
                n169 = call <vilib>:"NT Read Number.vi"("Name"=w261) -> ("Numeric"=w260:dbl)  [unwired: 9 in, 1 out]
                n170 = local write "Test Slider"(w260) -> ()
                n171 = property on="Test Slider" class="Slide (strict)"("Visible"=TRUE, "Scale.Maximum"=100.0 ("Scale.Range:Maximum")) -> ()  [unwired: 2 in, 2 out]
                n172 = property on="Test Ring" class="Ring (strict)"("Visible"=FALSE) -> ()  [unwired: 2 in, 2 out]
              }
            }
          }
        }
        n173 = property on="Progress" class="Clust (strict)"("Visible"=FALSE) -> ()  [unwired: 2 in, 2 out]
      }
      event "Test Name": Mouse Enter {
        # "Populate the ring with the list of tests"
        n174 = event-data() -> ()  [unwired: 1 in, 1 out]
        n175 = call <vilib>:"NT Read String Array.vi"("Name"="TestMode/TestList") -> ("String Array"=w269:string[])  [unwired: 9 in, 1 out]
        n176 = Build Array (concatenate)("Select the test to run...", w269) -> (w268:string[])
        n177 = property on="Test Name" class="Ring (strict)"("Strings []"=w268) -> ()  [unwired: 2 in, 2 out]
      }
      event "Test Name": Value Change {
        w271 = FALSE ("Visible")
        # "Tell the robot the test name to run"
        n178 = event-data() -> ("NewVal"=w275:u16)  [unwired: 1 in]
        n179 = property on="Test Name" class="Ring (strict)"() -> ("Strings []"=w276:string[])  [unwired: 2 in, 2 out]
        n180 = local write "Progress"(T6 {"Test Progress"=0, "Test Progress Text"=""} ("Progress")) -> ()
        n181 = Index Array(array=w276, index=w275) -> (element=w274:string)
        n182 = call <vilib>:"NT Write String.vi"("String"=w274, "Name"="TestMode/TestName") -> ()  [unwired: 9 in, 1 out]
        n183 = property on="Progress" class="Clust (strict)"("Visible"=TRUE) -> ()  [unwired: 2 in, 2 out]
        n184 = property on="Motor" class="Clust (strict)"("Visible"=w271) -> ()  [unwired: 2 in, 2 out]
        n185 = property on="Test Slider" class="Slide (strict)"("Visible"=w271) -> ()  [unwired: 2 in, 2 out]
        n186 = property on="On/Off" class="Bool (strict)"("Visible"=w271) -> ()  [unwired: 2 in, 2 out]
        n187 = property on="Rev/Fwd" class="Clust (strict)"("Visible"=w271) -> ()  [unwired: 2 in, 2 out]
        n188 = property on="Test Ring" class="Ring (strict)"("Visible"=w271) -> ()  [unwired: 2 in, 2 out]
      }
      event "Listbox": Double Click {
        # "Shift clears all"
        # "Update symbols on the listbox"
        n189 = event-data() -> ("PlatMods.Shift"=w279:bool, "Row"=w281:i32)  [unwired: 1 in]
        n190 = case shown="True" w279 {
          tunnel: w281 -> [w285 _]
          tunnel: 1 -> [w284 _]
          frame False {
            n191 = property on="Listbox" class="LstBox (strict)"() -> ("Item Symbols"=w283:i32[])  [unwired: 2 in, 2 out]
            n192 = Replace Array Subset(array=w283, new element=w284, index=w285) -> (w282:i32[])
            n193 = property on="Listbox" class="LstBox (strict)"("Item Symbols"=w282) -> ()  [unwired: 2 in, 2 out]
          }
          frame True {
            w286 = 0 ("Top Row")
            n194 = property on="Listbox" class="LstBox (strict)"() -> ("Number of Rows"=w288:u32)  [unwired: 2 in, 2 out]
            n195 = Initialize Array(0, w288) -> (w287:i32[])
            n196 = property on="Listbox" class="LstBox (strict)"("Top Row"=w286, "Value"=w286, "Item Symbols"=w287) -> ()  [unwired: 2 in, 2 out]
          }
        }
      }
      event "Listbox": Key Down {
        # "Update symbols on the listbox\nLeft and right keys check and uncheck"
        n197 = event-data() -> ("VKey"=w292:T18)  [unwired: 1 in]
        n198 = case shown="\"Left\", \"Right\"" w292 {
          selector: w292 -> [w297 _]
          tunnel: eventvkey."Left" ("VKey") -> [w295 _]
          frame "Left", "Right" {
            n199 = Equal?(x=w295, y=w297) -> (x = y?=w296:bool)
            n200 = Select(t=0, s=w296, f=1) -> (s? t:f=w298:i32)
            n201 = property on="Listbox" class="LstBox (strict)"() -> ("Item Symbols"=w301:i32[])  [unwired: 2 in, 2 out]
            n202 = Replace Array Subset(array=w301, new element=w298, index="Listbox") -> (w300:i32[])
            n203 = property on="Listbox" class="LstBox (strict)"("Item Symbols"=w300) -> ()  [unwired: 2 in, 2 out]
          }
          frame Default {
          }
        }
      }
      event "DB Camera Config": Value Change {
        # "Show or hide the cluster of controls, store in ini file"
        n204 = event-data() -> ("NewVal"=w305:bool)  [unwired: 1 in]
        n205 = case shown="False" w305 {
          tunnel: w304 -> [w314 _]
          tunnel: [w307 w325] -> w303
          tunnel: w302 -> [w306 w325]
          frame False {
            w321 = "Camera"
            w324 = FALSE ("Visible")
            n206 = local read "Camera Settings"() -> (w313:T2)
            n207 = Index Array(array=w314) -> (element=w317:cluster{string[]})  [unwired: 1 in]
            n208 = Unbundle(w313) -> ("Frame Rate"=w312:i32, "Compression"=w311:i32, "Size"=w315:u16)
            n209 = Unbundle(w317) -> (w316:string[])
            n210 = Index Array(array=w316, index=w315) -> (element=w310:string)
            n211 = call-poly <vilib>:"Write Key.vi"("section"=w321, "value"=w310, "key"="Size", "refnum"=w306) -> ("refnum out"=w323:T16)  [unwired: 2 in, 5 out]
            n212 = call-poly <vilib>:"Write Key.vi"("section"=w321, "value"=w312, "key"="FrameRate", "refnum"=w323) -> ("refnum out"=w322:T16)  [unwired: 1 in, 6 out]
            n213 = property on="Camera Settings" class="Clust (strict)"("Visible"=w324) -> ()  [unwired: 2 in, 2 out]
            n214 = local write "DB Camera Config"(w324) -> ()
            n215 = call-poly <vilib>:"Write Key.vi"("section"=w321, "value"=w311, "key"="Compression", "refnum"=w322) -> ("refnum out"=w308:T16)  [unwired: 1 in, 6 out]
            n216 = call <vilib>:"Close Config Data.vi"("refnum"=w308) -> ("file path"=w309:path)  [unwired: 2 in, 8 out]
            n217 = call <vilib>:"Open Config Data.vi"("configuration file path"=w309) -> ("refnum"=w307:T16)  [unwired: 8 in, 2 out]
          }
          frame True {
            n218 = property on="Camera Settings" class="Clust (strict)"("Visible"=TRUE) -> ()  [unwired: 2 in, 2 out]
          }
        }
      }
      event "Camera Settings": Value Change {
        # "Update summary string when any elements of DB camera change"
        n219 = event-data() -> ("NewVal"=w338:T2)  [unwired: 1 in]
        n220 = Index Array(array=w334) -> (element=w333:cluster{string[]})  [unwired: 1 in]
        n221 = Unbundle(w338) -> ("Frame Rate"=w329:i32, "Compression"=w328:i32, "Size"=w331:u16)
        n222 = Unbundle(w333) -> (w332:string[])
        n223 = Index Array(array=w332, index=w331) -> (element=w330:string)
        n224 = Format Into String(format string="%s   %dfps   %d%%", w330, w329, w328) -> (resulting string=w335:string)  [unwired: 2 in, 1 out]
        n225 = Build Array(w335) -> (w336:string[])
        n226 = property on="DB Camera Config" class="Bool (strict)"("Strings [4]"=w336) -> ()  [unwired: 2 in, 2 out]
      }
      event "Motor.Enable": Value Change {
        # "When the test mode otor enable helper is set, update that\ntree row item's value"
        n227 = event-data() -> ("NewVal"=w344:bool)  [unwired: 1 in]
        n228 = Unbundle("Motor") -> ("Value"=w343:dbl)  [unwired: 1 out]
        n229 = Select(t=w343, s=w344, f=0.0) -> (s? t:f=w341:dbl)
        n230 = call <vilib>:"NT Write Number.vi"("Numeric"=w341, "Name"=w340) -> ()  [unwired: 9 in, 1 out]
      }
      event "Test Slider": Value Change {
        # "When the test mode slider helper is set, update that\ntree row item's value"
        n231 = event-data() -> ("NewVal"=w347:dbl)  [unwired: 1 in]
        n232 = call <vilib>:"NT Write Number.vi"("Numeric"=w347, "Name"=w348) -> ()  [unwired: 9 in, 1 out]
      }
      event "On/Off": Value Change {
        # "When the test mode on/off helper value is set, update that\ntree row item's value"
        n233 = event-data() -> ("NewVal"=w352:bool)  [unwired: 1 in]
        n234 = Boolean To (0,1)(Boolean=w352) -> (0, 1=w351:i16)
        n235 = call <vilib>:"NT Write Number.vi"("Numeric"=w351, "Name"=w350) -> ()  [unwired: 9 in, 1 out]
      }
      event "Rev/Fwd": Value Change {
        # "When the test mode helper value for relays is set, update that\ntree row item's value"
        n236 = event-data() -> ("NewVal.Forward"=w360:bool, "NewVal.Reverse"=w359:bool)  [unwired: 1 in]
        n237 = Boolean To (0,1)(Boolean=w360) -> (0, 1=w356:i16)
        n238 = Boolean To (0,1)(Boolean=w359) -> (0, 1=w358:i16)
        n239 = Negate(x=w358) -> (-x=w357:i16)
        n240 = Add(x=w356, y=w357) -> (x+y=w355:i16)
        n241 = call <vilib>:"NT Write Number.vi"("Numeric"=w355, "Name"=w354) -> ()  [unwired: 9 in, 1 out]
      }
      event "Test Ring": Value Change {
        # "When a test mode helper value is selected from the ring,\nset the tree item's variable to the string value"
        n242 = event-data() -> ("NewVal"=w364:u16)  [unwired: 1 in]
        n243 = property on="Test Ring" class="Ring (strict)"() -> ("Strings []"=w365:string[])  [unwired: 2 in, 2 out]
        n244 = Index Array(array=w365, index=w364) -> (element=w363:string)
        n245 = call <vilib>:"NT Write String.vi"("String"=w363, "Name"=w362) -> ()  [unwired: 9 in, 1 out]
      }
      event "Rec Mode": Value Change {
        # "Update globals for recording mode and path to read log from.\nClear when logging and let NetworkTables set path for vision to\nuse."
        n246 = event-data() -> ("NewVal"=w375:enum32{"Stop", "Record", "Playback"})  [unwired: 1 in]
        n247 = global write "WPI_DashboardLogging Global.vi" "Logging Filename"(path "") -> ()
        n248 = case shown="\"Playback\"" w375 {
          tunnel: w374 -> [_ w377 w385]
          tunnel: [_ _ w384] -> w371
          tunnel: [_ _ w383] -> _
          tunnel: w369 -> [_ _ w381]
          tunnel: cluster{i32, i32} {-250, 170} -> [_ _ w380]
          tunnel: [_ _ T19 {"Image Size"=TRUE, "Image Type"=TRUE, "Pixel Value"=TRUE, "ROI Information"=TRUE, "Zoom Factor"=FALSE} ("Image Information Shown:All Elements")] -> w367
          tunnel: [_ _ TRUE ("Zoom Factor")] -> w366
          frame Default {
          }
          frame "Stop", "Record" {
            # "Place Window too"
            n249 = invoke class="VI" method="FP.Close"(reference=w377) -> (reference out=w376:refnum<vi>)  [unwired: 2 in, 2 out]
            n250 = invoke class="VI" method="Abort VI"(reference=w376) -> ()  [unwired: 2 in, 3 out]
          }
          frame "Playback" {
            n251 = call "Open Playback Panel.vi"("Offset"=w380, "DB VI Ref"=w381, "Playback in"=w385) -> ("Playback out"=w382:refnum<vi>)  [unwired: 8 in]
            n252 = register-events(w382) -> (reference out=w384:refnum<event-registration>, error out=w383:errorcluster)  [unwired: 2 in]
          }
        }
        n253 = global write "WPI_DashboardLogging Global.vi" "Recording"(w375) -> ()
        n254 = property on="Camera Image" class="ImageControl"("Image Information Shown"=w367, "Image Information Visible"=w366) -> ()  [unwired: 2 in, 2 out]
        n255 = call <vilib>:"WPI_DashboardNT Log FieldName Cache.vi"("Operation"=enum16{"Lookup/Add", "Index", "Clear"}."Clear") -> ()  [unwired: 8 in, 3 out]
      }
      event Panel Close {
        w386 = enum32{"Stop", "Record", "Playback"}."Stop" ("Rec Mode")
        # "Playback window has been closed, abort"
        n256 = event-data() -> ()  [unwired: 1 in, 4 out]
        n257 = local write "Rec Mode"(w386) -> ()
        n258 = global write "WPI_DashboardLogging Global.vi" "Recording"(w386) -> ()
      }
      event Panel Close {
        # "Abort playback window and ourself"
        n259 = event-data() -> ()  [unwired: 1 in, 4 out]
        n260 = invoke class="VI" method="FP.Close"(reference=w391) -> (reference out=w390:refnum<vi>)  [unwired: 2 in, 2 out]
        n261 = invoke class="VI" method="Abort VI"(reference=w390) -> (error out=w389:errorcluster)  [unwired: 2 in, 2 out]
        n262 = invoke class="VI" method="Abort VI"(error in=w389) -> ()  [unwired: 2 in, 3 out]
      }
      event "Vision": Value Change {
        # "Enable/Disable Compression slider.\nHW USB is hard-coded into the camera"
        n263 = event-data() -> ("NewVal"=w397:u16)  [unwired: 1 in]
        n264 = Equal?(x=w397, y=u32 2 ("milliseconds to wait")) -> (x = y?=w395:bool)
        n265 = Select(t=T20."Disabled and Grayed Out" ("Disabled"), s=w395, f=T20."Enabled" ("Disabled")) -> (s? t:f=w392:T20)
        n266 = property on="Compression" class="Slide (strict)"("DisabledEnum"=w392) -> ()  [unwired: 2 in, 2 out]
      }
    }
  }
  n267 = while {
    tunnel: w38 -> [w400]
    i -> [w403]
    stop <- FALSE stop-if-true
    n268 = Wait (ms)(milliseconds to wait=u32 100) -> ()  [unwired: 1 out]
    n269 = case shown="\"Playback\"" "Rec Mode" {
      tunnel: w403 -> [_ _ w418]
      tunnel: [u32 2829099 ("Base Color") u32 11141120 ("Target Color") w407] -> w399
      frame "Stop", Default {
        # "Reset the color, extra updates don't cost much"
      }
      frame "Record" {
      }
      frame "Playback" {
        # "Playback"
        n270 = Quotient & Remainder(x=w418, y=u32 50 ("milliseconds to wait")) -> (x-y*floor(x/y)=w414:u32)  [unwired: 1 out]
        n271 = Divide(x=w414, y=u32 50 ("milliseconds to wait")) -> (x/y=w411:dbl)
        n272 = Multiply(x=6.283185307179586, y=w411) -> (x*y=w416:dbl)
        n273 = Sine(x=w416) -> (sin(x)=w415:dbl)
        n274 = Absolute Value(x=w415) -> (abs(x)=w408:dbl)
        n275 = call "Interpolate RGB Color.vi"("Proportion"=w408, "Target Color"=u32 30976, "Base Color"=u32 2829099) -> ("Result Color"=w407:u32)  [unwired: 8 in]
      }
    }
    n276 = property class="Pane"(reference=w400, "PaneColor"=w399) -> ()  [unwired: 1 in, 2 out]
  }
  n277 = TCP Create Listener(10:u16 1741 ("timeout ms (25000)")) -> (3:w1:refnum<k5>)  [unwired: 4 in, 2 out]
  n278 = while {
    tunnel: w1 -> [w420]
    stop <- FALSE stop-if-true
    n279 = TCP Wait On Listener(11:w420) -> (4:w419:refnum<k5>)  [unwired: 3 in, 4 out]
    n280 = local write "TCP"(w419) -> ()
  }
  n281 = property on="On/Off" class="Bool (strict)"("Visible"=w6) -> ()  [unwired: 2 in, 2 out]
  n282 = property on="Motor" class="Clust (strict)"("Visible"=w6) -> ()  [unwired: 2 in, 2 out]
  n283 = property on="Progress" class="Clust (strict)"("Visible"=w6) -> ()  [unwired: 2 in, 2 out]
  n284 = property on="Test Ring" class="Ring (strict)"("Visible"=w6) -> ()  [unwired: 2 in, 2 out]
  n285 = property on="Rev/Fwd" class="Clust (strict)"("Visible"=w6) -> ()  [unwired: 2 in, 2 out]
  n286 = property on="Camera Settings" class="Clust (strict)"("Visible"=w6) -> ()  [unwired: 2 in, 2 out]
  n287 = local write "DB Camera Config"(w6) -> ()
  n288 = global write "WPI_DashboardLogging Global.vi" "Recording"(w32) -> ()
  n289 = local write "Rec Mode"(w32) -> ()
